vi "Identify.vi"(8 "error in (no error)":errorcluster, 11 "Harmonics in":refnum<class "Harmonics.lvclass">) -> (0 "error out":errorcluster, 2 "Plugin is Valid":bool, 3 "Harmonics out":refnum<class "Harmonics.lvclass">)   [LabVIEW 2018, in "Harmonics.lvlib" / "Harmonics.lvclass"]
uses:
  Harmonics.lvclass
  C:/Sequence Automation/Plugins/Measurement Interface.lvlibp/Measurement Interface.lvclass
  Plugins/Measurement Interface.lvlibp/Private Methods/Measurement Definition Entry/Read Measurement Definition Entry.vi
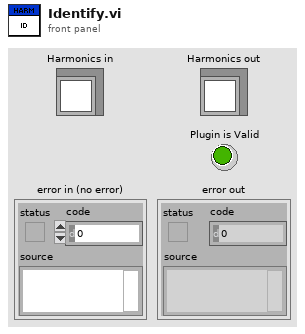
[diagram p1: front panel]
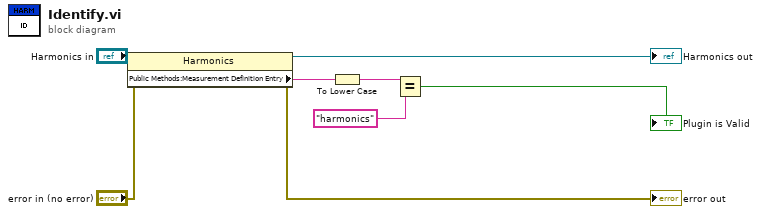
[diagram p0: block diagram]
diagram:
  n1 = property class="Harmonics"(reference="Harmonics in", error in="error in (no error)") -> (reference out=→"Harmonics out":refnum<class "Harmonics.lvclass">, error out=→"error out":errorcluster, "Public Methods:Measurement Definition Entry"=w4:string)
  n2 = To Lower Case(string=w4) -> (all lower case string=w3:string)
  n3 = Equal?(x=w3, y="harmonics" ("Entry Name")) -> (x = y?=→"Plugin is Valid":bool)
